vi "Lookup Channel Indices.vi"(8 "error in (no error)":errorcluster, 11 "System Health Module in":refnum<class "System Health Module.lvclass">) -> (0 "error out":errorcluster, 3 "System Health Module out":refnum<class "System Health Module.lvclass">)   [LabVIEW 2020, in "Volatus.lvlib" / "System Health Module.lvclass"]
uses:
  System Health Module.lvclass
  C:/dev/lv20CE/relink/lv-volatus/Volatus/Module/Module.lvclass
  Module/Module.lvclass/Module.ctl
  VolatusConfig/VolatusConfigElement/VolatusConfigElement.lvclass/VolatusConfigElement.ctl
  System Health Module.lvclass/System Health Module.ctl
  Module/Config.vi
  VolatusConfig/VolatusConfigElement/Element.vi
  VolatusConfig/Group/Group.lvclass
  C:/dev/lv20CE/relink/lv-volatus/VolatusConfig/VolatusConfigElement/VolatusConfigElement.lvclass
  lv-cdm/CDM-Config/Config Element/Owner.vi
  lv-cdm/CDM-Config/Config Manager/Lookup Descendant.vi
  VolatusConfig/Task/Task.lvclass
  Module/Module.lvclass
  VolatusConfig/VolatusConfigElement/VolatusConfigElement.lvclass
  lv-cdm/CDM-Config/Config Element/Config Element.lvclass
  lv-cdm/CDM-Config/Config Filter/Config Lookup.lvclass
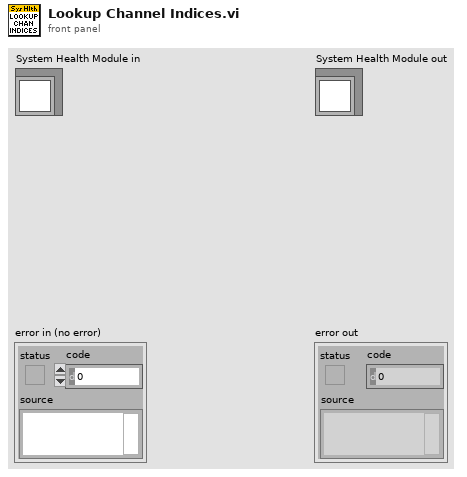
[diagram p1: front panel]
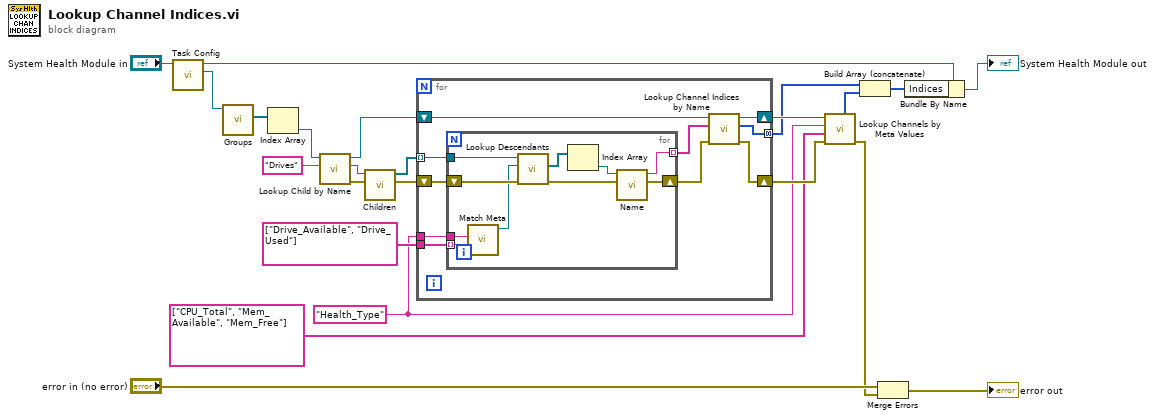
[diagram p0: block diagram]
diagram:
  w8 = "Health_Type" ("Name")
  n1 = call "Task Config.vi"("Module in"="System Health Module in") -> ("Task Config"=w13:refnum<class "Task.lvclass">, "Module out"=w19:refnum<class "System Health Module.lvclass">)  [unwired: 8 in, 1 out]
  n2 = call "Groups.vi"("Task in"=w13) -> ("Groups"=w12:refnum<class "Group.lvclass">[])  [unwired: 8 in, 2 out]
  n3 = Index Array(array=w12) -> (element=w11:refnum<class "Group.lvclass">)  [unwired: 1 in]
  n4 = call "Lookup Child by Name.vi"("Child Name"="Drives", "VolatusConfigElement in"=w11) -> ("error out"=w17:errorcluster, "Child"=w16:refnum<class "Config Element.lvclass">, "VolatusConfigElement out"=w10:refnum<class "Group.lvclass">)  [unwired: 6 in, 1 out]
  n5 = call "Children.vi"("error in (no error)"=w17, "Config Element in"=w16) -> ("error out"=w15:errorcluster, "Elements"=w14:refnum<class "Config Element.lvclass">[])  [unwired: 8 in]
  n6 = for {
    tunnel: string[] ["Drive_Available", "Drive_Used"] -> [w33]
    shift-right: [w26] -> w23
    shift-left: w15 -> [w31]
    tunnel: w14 -> [w30] mode=indexing
    tunnel: w8 -> [w32]
    tunnel: [w25] -> w6 mode=concatenating
    shift-right: [w24] -> w9
    shift-left: w10 -> [w29]
    n7 = for {
      tunnel: w33 -> [w43] mode=indexing
      tunnel: w32 -> [w42]
      tunnel: w30 -> [w40]
      shift-right: [w35] -> w27
      shift-left: w31 -> [w41]
      tunnel: [w34] -> w28 mode=indexing
      n8 = call "Match Meta.vi"("Value (Any)"=w43, "Name"=w42) -> ("Config Lookup out"=w39:refnum<class "Config Lookup.lvclass">)  [unwired: 8 in, 1 out]
      n9 = call "Lookup Descendants.vi"("error in (no error)"=w41, "Lookup"=w39, "Config Element in"=w40) -> ("error out"=w36:errorcluster, "Descendants"=w38:refnum<class "Config Element.lvclass">[])  [unwired: 6 in, 1 out]
      n10 = Index Array(array=w38) -> (element=w37:refnum<class "Config Element.lvclass">)  [unwired: 1 in]
      n11 = call "Name.vi"("error in (no error)"=w36, "Config Element in"=w37) -> ("error out"=w35:errorcluster, "Name"=w34:string)  [unwired: 8 in]
    }
    n12 = call "Lookup Channel Indices by Name.vi"("error in (no error)"=w27, "Channel Names"=w28, "Group in"=w29) -> ("error out"=w26:errorcluster, "Indices"=w25:i32[], "Group out"=w24:refnum<class "Group.lvclass">)  [unwired: 6 in]
  }
  n13 = call "Lookup Channels by Meta Values.vi"("error in (no error)"=w23, "Meta Values"=string[] ["CPU_Total", "Mem_Available", "Mem_Free"], "Meta Name"=w8, "Group in"=w9) -> ("error out"=w1:errorcluster, "Indices"=w5:i32[])  [unwired: 4 in, 2 out]
  n14 = Build Array (concatenate)(w6, w5) -> (w3:i32[])
  n15 = Merge Errors("error in (no error)", w1) -> (→"error out":errorcluster)
  n16 = Bundle By Name(cluster=w19, "Indices"=w3) -> (→"System Health Module out":refnum<class "System Health Module.lvclass">)
